vi "S8300E_RTC_PC_Compare.vi"() -> ()   [LabVIEW 2011]
uses:
  Instance          11 29Saved   Mojo_RTC_SFCS_Compare .vi
  Instance           1 29Saved   Mojo_RTC_SFCS_Compare .vi
  Instance           4 29Saved   Mojo_RTC_SFCS_Compare .vi
  Instance           2 29Saved   Mojo_RTC_SFCS_Compare .vi
panel:
  out "log":string
  out "Temp Log":string
  out "PC_Date_Time":string="15:37"
  out "Tolerance sec":string
  out "UUT sec":i32
  out "UUT min":i32
  out "UUT hour":i32
  out "UUT Day":i32
  out "UUT  Month":i32
  out "UUT Year":i32
  out "UUT-DateTime":string
  out "VISA resource name out":refnum<visa-resource-name>
  out "Start Time":u32
  out "Tolerance_sec_gap":dbl
  out "TimeGap(sec)":dbl format="%#_8f"
  out "sec":i32
  out "minute":i32
  out "hour":i32
  out "day":i32
  out "month":i32
  out "year":i32
  out "PC_Time":string
  out "PC_DATE_STRING":string
  out "STAGE":string
  out "SFCS_IP":string
  # "Error Code:RTC\nError Code:UART"
  # "PC時間與S8300E 時間比較\nPC Time compare to S8300E RTC Time"
  # "2015-6-12"
  # "COM9, Baud 115200"
  # "PC Time:"
  # "UUT-Date-Time:"
  # "Formula :TimeGap=SFCS Time-UUT Time"
  # "<"
  # "Pass Criteria"
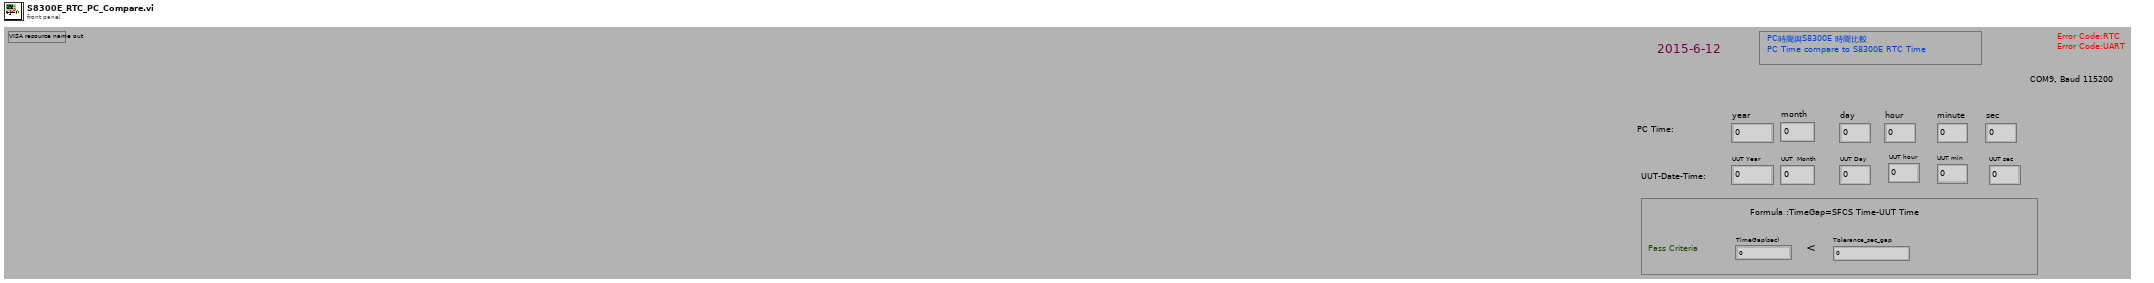
[diagram p1: front panel]
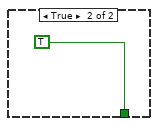
[diagram p5: hidden frame]
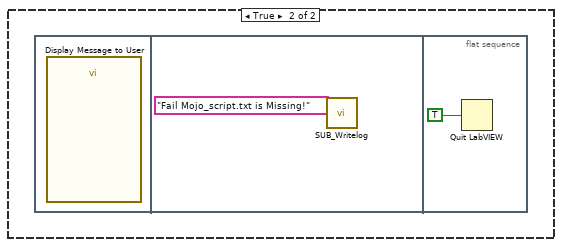
[diagram p7: hidden frame]
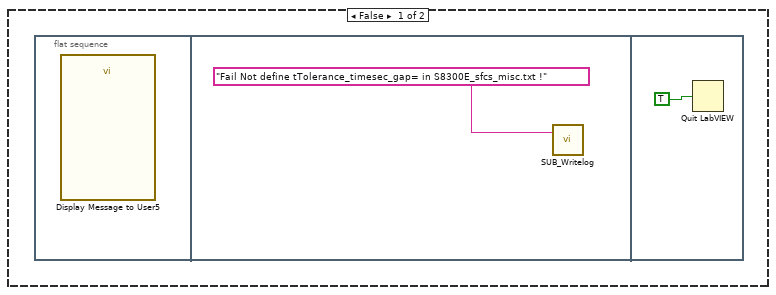
[diagram p8: hidden frame]
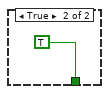
[diagram p11: hidden frame]
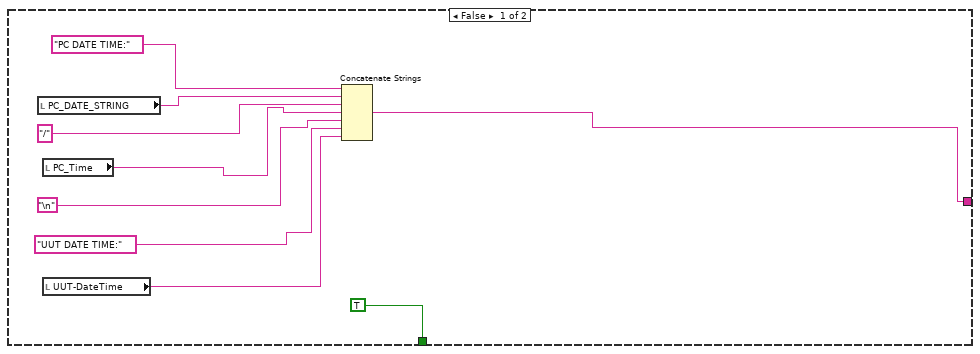
[diagram p12: hidden frame]
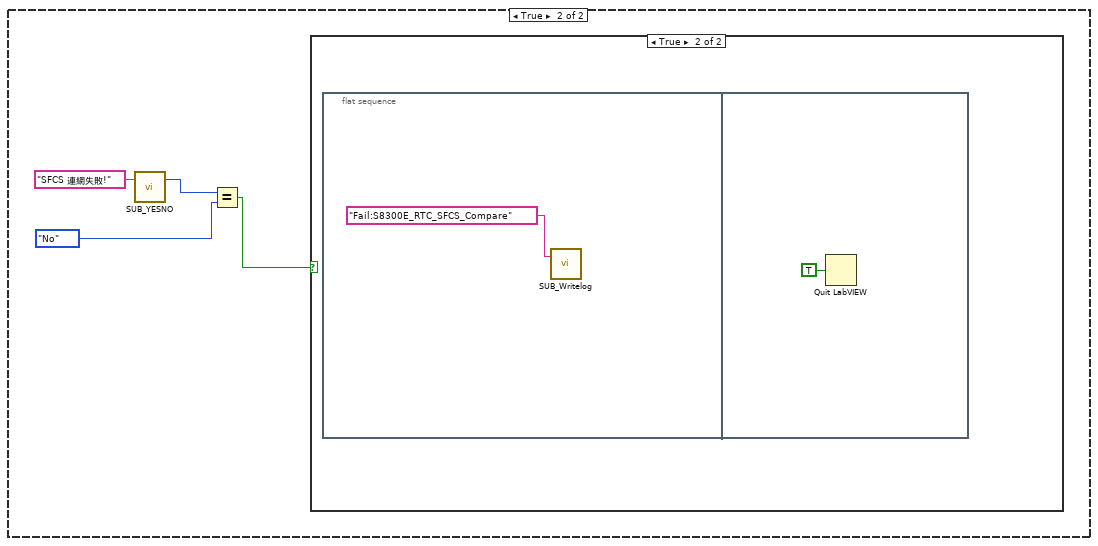
[diagram p14: hidden frame]
diagram:
  n1 = flat-sequence {
    tunnel: [w34] -> w2
    tunnel: w2 -> [w57]
    tunnel: [w57] -> w1
    tunnel: w1 -> [w65]
    frame #0 {
      n2 = Tick Count (ms)() -> (millisecond timer value=→"Start Time":u32)
    }
    frame #1 {
      n3 = call "SUB_COM1_CLOSE.vi"("VISA resource name"=refnum<visa-resource-name> "COM9") -> ()  [unwired: 3 in]
    }
    frame #2 {
      n4 = case shown="True" TRUE {
        frame False {
        }
        frame True {
          n5 = call "SUB_COM9_INIT.vi"("baud rate"=u32 115200) -> ("VISA resource name out"=w9:refnum<visa-resource-name>)  [unwired: 1 in, 1 out]
          "VISA resource name out" <- w9
          n6 = call "SUB_COM1Wrt.vi"("VISA resource name"=w9, "write buffer"="\r") -> ("duplicate VISA resource name"=w6:refnum<visa-resource-name>)  [unwired: 1 in, 1 out]
          n7 = call "SUB_ContinueCom1Read.vi"("Numeric"=1200, "duplicate VISA resource name 2"=w6) -> ()  [unwired: 1 in, 3 out]
        }
      }
    }
    frame #3 {
      n8 = case shown="True" TRUE {
        frame False {
        }
        frame True {
          n9 = while {
            stop <- w19 stop-if-true
            n10 = local read "VISA resource name out"() -> (w18:refnum<visa-resource-name>)
            n11 = Tick Count (ms)() -> (millisecond timer value=w13:u32)
            n12 = call "SUB_COM1Wrt.vi"("VISA resource name"=w18, "write buffer"="\r") -> ("duplicate VISA resource name"=w14:refnum<visa-resource-name>)  [unwired: 1 in, 1 out]
            n13 = call "SUB_READ_COM1_FindString_timeout.vi"("Find this String"="S8300E", "Timeout Seccond"=2.0, "Begin time"=w13, "duplicate VISA resource name 2"=w14) -> ("Output String"=w16:string, "Found String"=w15:bool)  [unwired: 1 in, 1 out]
            n14 = case shown="False" w15 {
              tunnel: w16 -> [w25 _]
              tunnel: [w21 TRUE] -> w19
              frame False {
                n15 = call "SUB_YESNO.vi"("Debug View"=w25, "Status"="UART無正確反應!需有S8300E字串") -> ("yes/no"=w24:enum32{"No Selection", "Yes", "No", "None"})  [unwired: 1 in]
                n16 = Equal?(x=w24, y=enum32{"No Selection", "Yes", "No", "None"}."No") -> (x = y?=w22:bool)
                n17 = case shown="True" w22 {
                  tunnel: [_ w27] -> w21
                  frame False {
                  }
                  frame True {
                    n18 = flat-sequence {
                      tunnel: [w31] -> w27
                      frame #0 {
                        n19 = call "SUB_Writelog.vi"("Pass/Fail"="Fail:S8300E_RTC_SFCS_Compare") -> ()  [unwired: 2 in]
                      }
                      frame #1 {
                        n20 = call "SUB_SFCS_SendResult.vi"("ErrorCode"="UART", "PASS_Fail (1/0)"=i8 0) -> ()  [unwired: 1 out]
                      }
                      frame #2 {
                        w31 = TRUE ("quit? (T)")
                        n21 = Quit LabVIEW(quit? (T)=w31) -> ()
                      }
                    }
                  }
                }
              }
              frame True {
              }
            }
          }
        }
      }
    }
    frame #4 {
      n22 = call "SUB_Read_specifFile.vi"("name or relative path"="S8300E_sfcs_misc.txt" ("Script FileName")) -> ("error out"=w37:errorcluster, "text"=w34:string)  [unwired: 1 in]
      n23 = Unbundle By Name(w37) -> ("code"=w36:i32)
      n24 = Not Equal To 0?(x=w36) -> (x != 0?=w35:bool)
      n25 = case shown="False" w35 {
        tunnel: w34 -> [w38 _]
        frame False {
          n26 = flat-sequence {
            tunnel: w38 -> [w44]
            frame #0 {
              n27 = To Upper Case(1:"SFCS_IP=" ("string")) -> (0:w48:string)
              n28 = To Upper Case(1:w44) -> (0:w49:string)
              n29 = call <vilib>:"Trim Whitespace.vi"("string"=w48) -> ("trimmed string"=w46:string)  [unwired: 1 in]
              n30 = call <vilib>:"Trim Whitespace.vi"("string"=w49) -> ("trimmed string"=w45:string)  [unwired: 1 in]
              n31 = Match Pattern(string=w45, regular expression=w46) -> (after substring=w43:string)  [unwired: 1 in, 3 out]
              n32 = Match Pattern(string=w43, regular expression=";") -> (before substring=w41:string)  [unwired: 1 in, 3 out]
              "SFCS_IP" <- w41
              n33 = Equal?(x=w41, y="") -> (x = y?=w39:bool)
              n34 = case shown="True" w39 {
                frame False {
                }
                frame True {
                  n35 = flat-sequence {
                    frame #0 {
                      n36 = call "Display Message to User2"() -> ()  [unwired: 10 in, 2 out]
                    }
                    frame #1 {
                      n37 = call "SUB_Writelog.vi"("Pass/Fail"="Fail Not Found SFCS_IP=\"xx.xx.xx.xx\" in S8300E_sfcs_misc.txt !") -> ()  [unwired: 2 in]
                    }
                    frame #2 {
                      n38 = Quit LabVIEW(quit? (T)=TRUE) -> ()
                    }
                  }
                }
              }
            }
          }
        }
        frame True {
          n39 = flat-sequence {
            frame #0 {
              n40 = call "Display Message to User"() -> ()  [unwired: 10 in, 2 out]
            }
            frame #1 {
              n41 = call "SUB_Writelog.vi"("Pass/Fail"="Fail Mojo_script.txt is Missing!") -> ()  [unwired: 2 in]
            }
            frame #2 {
              n42 = Quit LabVIEW(quit? (T)=TRUE) -> ()
            }
          }
        }
      }
    }
    frame #5 {
      n43 = call "SUB_FindSpecificString.vi"("Find this String"="Tolerance_timesec_gap=", "String data"=w57) -> ("before \"; \" string"=w54:string, "Found"=w55:bool)  [unwired: 2 in]
      n44 = case shown="True" w55 {
        tunnel: w54 -> [_ w61]
        frame False {
          n45 = flat-sequence {
            frame #0 {
              n46 = call "Display Message to User5"() -> ()  [unwired: 10 in, 2 out]
            }
            frame #1 {
              n47 = call "SUB_Writelog.vi"("Pass/Fail"="Fail Not define tTolerance_timesec_gap= in S8300E_sfcs_misc.txt !") -> ()  [unwired: 2 in]
            }
            frame #2 {
              n48 = Quit LabVIEW(quit? (T)=TRUE) -> ()
            }
          }
        }
        frame True {
          n49 = Fract/Exp String To Number(string=w61) -> (number=→"Tolerance_sec_gap":dbl)  [unwired: 3 in, 1 out]
          "Tolerance sec" <- w61
        }
      }
    }
    frame #6 {
      n50 = To Upper Case(1:"SFCS_STAGE=" ("string")) -> (0:w71:string)
      n51 = To Upper Case(1:w65) -> (0:w72:string)
      n52 = call <vilib>:"Trim Whitespace.vi"("string"=w71) -> ("trimmed string"=w70:string)  [unwired: 1 in]
      n53 = call <vilib>:"Trim Whitespace.vi"("string"=w72) -> ("trimmed string"=w69:string)  [unwired: 1 in]
      n54 = Match Pattern(string=w69, regular expression=w70) -> (after substring=w68:string)  [unwired: 1 in, 3 out]
      n55 = Match Pattern(string=w68, regular expression=";") -> (before substring=w64:string)  [unwired: 1 in, 3 out]
      "STAGE" <- w64
      n56 = Not Equal?(x=w64, y="") -> (x != y?=w62:bool)
      n57 = case shown="False" w62 {
        frame False {
          n58 = flat-sequence {
            frame #0 {
              n59 = call "Display Message to User4"() -> ()  [unwired: 10 in, 2 out]
            }
            frame #1 {
              n60 = call "SUB_Writelog.vi"("Pass/Fail"="Fail :Stage  not define in script file!") -> ()  [unwired: 2 in]
            }
            frame #2 {
              n61 = Quit LabVIEW(quit? (T)=TRUE) -> ()
            }
          }
        }
        frame True {
        }
      }
    }
    frame #7 {
      n62 = while {
        stop <- w80 stop-if-true
        n63 = Concatenate Strings("./rtc.sh -r" ("string"), "\r") -> (w86:string)
        n64 = Tick Count (ms)() -> (millisecond timer value=w76:u32)
        n65 = local read "VISA resource name out"() -> (w84:refnum<visa-resource-name>)
        n66 = call "SUB_COM1Wrt.vi"("VISA resource name"=w84, "write buffer"=w86) -> ("duplicate VISA resource name"=w77:refnum<visa-resource-name>)  [unwired: 1 in, 1 out]
        n67 = call "SUB_READ_COM1_FindString_timeout.vi"("Find this String"="PASSED=", "Timeout Seccond"=3.0, "Begin time"=w76, "duplicate VISA resource name 2"=w77) -> ("Output String"=w79:string)  [unwired: 1 in, 2 out]
        n68 = call "SUB_FindSpecificString.vi"("Find this String"="PASSED=", "String data"=w79) -> ("before \"; \" string"=→"UUT-DateTime":string, "Found"=w81:bool)  [unwired: 2 in]
        n69 = case shown="False" w81 {
          tunnel: w79 -> [w91 _]
          tunnel: [_ TRUE] -> w80
          frame False {
            n70 = call "SUB_YESNO.vi"("Debug View"=w91, "Status"="無法取得UUT RTC Time") -> ("yes/no"=w90:enum32{"No Selection", "Yes", "No", "None"})  [unwired: 1 in]
            n71 = Equal?(x=w90, y=enum32{"No Selection", "Yes", "No", "None"}."No") -> (x = y?=w88:bool)
            n72 = case shown="True" w88 {
              frame False {
              }
              frame True {
                n73 = flat-sequence {
                  frame #0 {
                    n74 = call "SUB_Writelog.vi"("Pass/Fail"="Fail:S8300E_RTC_SFCS_Compare") -> ()  [unwired: 2 in]
                  }
                  frame #1 {
                    n75 = call "SUB_SFCS_SendResult.vi"("ErrorCode"="RTC", "PASS_Fail (1/0)"=i8 0) -> ()  [unwired: 1 out]
                  }
                  frame #2 {
                    n76 = Quit LabVIEW(quit? (T)=TRUE) -> ()
                  }
                }
              }
            }
          }
          frame True {
          }
        }
      }
    }
    frame #8 {
      n77 = local read "UUT-DateTime"() -> (w104:string)
      n78 = call "SUB_UUT_DatTime_Display.vi"("UUT_DateTime_input"=w104) -> ("UUT sec"=→"UUT sec":i32, "UUT min"=→"UUT min":i32, "UUT hour"=→"UUT hour":i32, "UUT Day"=→"UUT Day":i32, "UUT  Month"=→"UUT  Month":i32, "UUT Year"=→"UUT Year":i32)
    }
    frame #9 {
      n79 = while {
        shift-right: [w109] -> w105
        shift-left: "" -> [w107]
        stop <- w111 stop-if-true
        n80 = call "SUB_GETDateTime_String.vi"() -> ("date/time string"=w110:string)  [unwired: 3 in]
        "PC_Date_Time" <- w110
        n81 = To Upper Case(1:"FAIL" ("string")) -> (0:w118:string)
        n82 = To Upper Case(1:"NG" ("string")) -> (0:w126:string)
        n83 = To Upper Case(1:w110) -> (0:w127:string)
        n84 = call <vilib>:"Trim Whitespace.vi"("string"=w118) -> ("trimmed string"=w115:string)  [unwired: 1 in]
        n85 = call <vilib>:"Trim Whitespace.vi"("string"=w126) -> ("trimmed string"=w123:string)  [unwired: 1 in]
        n86 = call <vilib>:"Trim Whitespace.vi"("string"=w127) -> ("trimmed string"=w119:string)  [unwired: 1 in]
        n87 = Match Pattern(string=w110, regular expression=" ") -> (before substring=w121:string, after substring=w120:string)  [unwired: 1 in, 2 out]
        n88 = Match Pattern(string=w119, regular expression=w123) -> (match substring=w124:string)  [unwired: 1 in, 3 out]
        n89 = Match Pattern(string=w119, regular expression=w115) -> (match substring=w116:string)  [unwired: 1 in, 3 out]
        n90 = Equal?(x=w116, y=w115) -> (x = y?=w113:bool)
        n91 = Equal?(x=w124, y=w123) -> (x = y?=w114:bool)
        n92 = Or(x=w114, y=w113) -> (x .or. y?=w112:bool)
        n93 = case shown="False" w112 {
          tunnel: w121 -> [w141 _]
          tunnel: w120 -> [w140 _]
          tunnel: [w135 _] -> w111
          tunnel: [w128 _] -> w108
          frame False {
            n94 = flat-sequence {
              tunnel: w141 -> [w144]
              tunnel: w140 -> [w142]
              tunnel: [w148] -> w133
              tunnel: [w147] -> w131
              tunnel: [w146] -> w129
              tunnel: [w166] -> w139
              tunnel: [w165] -> w138
              tunnel: [w164] -> w137
              tunnel: [w163] -> w134
              tunnel: w133 -> [w163]
              tunnel: [w162] -> w132
              tunnel: w131 -> [w162]
              tunnel: [w161] -> w130
              tunnel: w129 -> [w161]
              tunnel: w139 -> [w181]
              tunnel: w138 -> [w180]
              tunnel: w137 -> [w179]
              tunnel: [w186] -> w136
              tunnel: w134 -> [w184]
              tunnel: w132 -> [w183]
              tunnel: w130 -> [w182]
              tunnel: w136 -> [w191]
              tunnel: [w188] -> w135
              tunnel: [w187] -> w128
              frame #0 {
                n95 = call <vilib>:"Trim Whitespace.vi"("string"=w144) -> ("trimmed string"=→"PC_DATE_STRING":string)  [unwired: 1 in]
                n96 = call <vilib>:"Trim Whitespace.vi"("string"=w142) -> ("trimmed string"=→"PC_Time":string)  [unwired: 1 in]
              }
              frame #1 {
                w155 = "/" ("regular expression")
                n97 = local read "PC_DATE_STRING"() -> (w160:string)
                n98 = Match Pattern(string=w160, regular expression=w155) -> (before substring=w159:string, after substring=w156:string)  [unwired: 1 in, 2 out]
                n99 = Match Pattern(string=w156, regular expression=w155) -> (before substring=w152:string, after substring=w150:string)  [unwired: 1 in, 2 out]
                n100 = call <vilib>:"Trim Whitespace.vi"("string"=w159) -> ("trimmed string"=w158:string)  [unwired: 1 in]
                n101 = To Upper Case(1:w158) -> (0:w157:string)
                n102 = call <vilib>:"Trim Whitespace.vi"("string"=w150) -> ("trimmed string"=w151:string)  [unwired: 1 in]
                n103 = call <vilib>:"Trim Whitespace.vi"("string"=w152) -> ("trimmed string"=w154:string)  [unwired: 1 in]
                n104 = To Upper Case(1:w151) -> (0:w149:string)
                n105 = To Upper Case(1:w154) -> (0:w153:string)
                n106 = Decimal String To Number(string=w157) -> (number=w148:i32)  [unwired: 2 in, 1 out]
                "year" <- w148
                n107 = Decimal String To Number(string=w149) -> (number=w146:i32)  [unwired: 2 in, 1 out]
                "day" <- w146
                n108 = Decimal String To Number(string=w153) -> (number=w147:i32)  [unwired: 2 in, 1 out]
                "month" <- w147
              }
              frame #2 {
                w174 = ":" ("regular expression")
                n109 = local read "PC_Time"() -> (w167:string)
                n110 = Match Pattern(string=w167, regular expression=w174) -> (before substring=w178:string, after substring=w175:string)  [unwired: 1 in, 2 out]
                n111 = Match Pattern(string=w175, regular expression=w174) -> (before substring=w171:string, after substring=w169:string)  [unwired: 1 in, 2 out]
                n112 = call <vilib>:"Trim Whitespace.vi"("string"=w178) -> ("trimmed string"=w177:string)  [unwired: 1 in]
                n113 = To Upper Case(1:w177) -> (0:w176:string)
                n114 = call <vilib>:"Trim Whitespace.vi"("string"=w169) -> ("trimmed string"=w170:string)  [unwired: 1 in]
                n115 = call <vilib>:"Trim Whitespace.vi"("string"=w171) -> ("trimmed string"=w173:string)  [unwired: 1 in]
                n116 = To Upper Case(1:w170) -> (0:w168:string)
                n117 = To Upper Case(1:w173) -> (0:w172:string)
                n118 = Decimal String To Number(string=w176) -> (number=w164:i32)  [unwired: 2 in, 1 out]
                "hour" <- w164
                n119 = Decimal String To Number(string=w168) -> (number=w166:i32)  [unwired: 2 in, 1 out]
                "sec" <- w166
                n120 = Decimal String To Number(string=w172) -> (number=w165:i32)  [unwired: 2 in, 1 out]
                "minute" <- w165
              }
              frame #3 {
                n121 = local read "UUT-DateTime"() -> (w185:string)
                n122 = call "SUB_TimeGAP_SFCS_RTC.vi"("SFCS year"=w184, "UUT_DateTime_input"=w185, "SFCS month"=w183, "SFCS day"=w182, "SFCS hour"=w179, "SFCS minute"=w180, "SFCS second"=w181) -> ("TimeGap(sec)"=w186:dbl)
                "TimeGap(sec)" <- w186
              }
              frame #4 {
                n123 = local read "Tolerance_sec_gap"() -> (w190:dbl)
                n124 = Greater?(x=w191, y=w190) -> (0:w189:bool)
                n125 = case shown="True" w189 {
                  tunnel: [TRUE _] -> w188
                  tunnel: [w192 w201] -> w187
                  frame False {
                    n126 = local read "PC_DATE_STRING"() -> (w198:string)
                    n127 = local read "PC_Time"() -> (w196:string)
                    n128 = local read "UUT-DateTime"() -> (w193:string)
                    n129 = Concatenate Strings("PC DATE TIME:" ("string"), w198, "/" ("string"), w196, "\n", "UUT DATE TIME:" ("string"), w193) -> (w192:string)
                  }
                  frame True {
                    n130 = local read "TimeGap(sec)"() -> (w213:dbl)
                    n131 = local read "Tolerance sec"() -> (w208:string)
                    n132 = Number To Fractional String(number=w213) -> (F-format string=w211:string)  [unwired: 3 in]
                    n133 = Concatenate Strings("Failed:TimeGap 需小於Tolerance Gap", "\n") -> (w204:string)
                    n134 = Concatenate Strings("目前TimeGap=" ("string"), w211, "\n", "目前ToleranceGap=" ("string"), w208) -> (w203:string)
                    n135 = call "SUB_YESNO.vi"("Debug View"=w203, "Status"=w204) -> ("yes/no"=w207:enum32{"No Selection", "Yes", "No", "None"})  [unwired: 1 in]
                    n136 = Concatenate Strings(w204, w203) -> (w202:string)
                    n137 = Equal?(x=w207, y=enum32{"No Selection", "Yes", "No", "None"}."No") -> (x = y?=w205:bool)
                    n138 = case shown="True" w205 {
                      tunnel: [w216 w217] -> w201
                      tunnel: w202 -> [w216 w217]
                      frame False {
                      }
                      frame True {
                        n139 = flat-sequence {
                          frame #0 {
                            n140 = local read "Temp Log"() -> (w218:string)
                            n141 = Concatenate Strings("Fail:S8300E_RTC_SFCS_Compare" ("Pass/Fail"), "\n", w218) -> (w221:string)
                            n142 = call "SUB_Writelog.vi"("Pass/Fail"=w221) -> ()  [unwired: 2 in]
                          }
                          frame #1 {
                            n143 = call "SUB_SFCS_SendResult.vi"("ErrorCode"="RTC", "PASS_Fail (1/0)"=i8 0) -> ()  [unwired: 1 out]
                          }
                          frame #2 {
                            n144 = Quit LabVIEW(quit? (T)=TRUE) -> ()
                          }
                        }
                      }
                    }
                  }
                }
              }
            }
          }
          frame True {
            n145 = call "SUB_YESNO.vi"("Status"="SFCS 連網失敗!") -> ("yes/no"=w227:enum32{"No Selection", "Yes", "No", "None"})  [unwired: 2 in]
            n146 = Equal?(x=w227, y=enum32{"No Selection", "Yes", "No", "None"}."No") -> (x = y?=w225:bool)
            n147 = case shown="True" w225 {
              frame False {
              }
              frame True {
                n148 = flat-sequence {
                  frame #0 {
                    n149 = call "SUB_Writelog.vi"("Pass/Fail"="Fail:S8300E_RTC_SFCS_Compare") -> ()  [unwired: 2 in]
                  }
                  frame #1 {
                    n150 = Quit LabVIEW(quit? (T)=TRUE) -> ()
                  }
                }
              }
            }
          }
        }
        n151 = Concatenate Strings(w107, w108) -> (w109:string)
        "Temp Log" <- w109
      }
      "log" <- w105
    }
    frame #10 {
      n152 = call "SUB_COM1_CLOSE.vi"("VISA resource name"=refnum<visa-resource-name> "COM9") -> ()  [unwired: 3 in]
    }
    frame #11 {
      w237 = "***Not Good ***" ("replace string (\"\")")
      w233 = "\r"
      n153 = local read "PC_Date_Time"() -> (w241:string)
      n154 = local read "TimeGap(sec)"() -> (w244:dbl)
      n155 = local read "log"() -> (w232:string)
      n156 = local read "UUT-DateTime"() -> (w246:string)
      n157 = Tick Count (ms)() -> (millisecond timer value=w250:u32)
      n158 = local read "Start Time"() -> (w249:u32)
      n159 = call "SUB_CAL_TESTTIME.vi"("Test Item name"="S8300E_RTC_SFCS_Compare", "Stop tick time"=w250, "Start tick time"=w249) -> ("Test Time output"=w242:string)  [unwired: 2 in]
      n160 = Number To Fractional String(number=w244) -> (F-format string=w243:string)  [unwired: 3 in]
      n161 = Concatenate Strings("Pass :S8300E_RTC_SFCS_Compare" ("Pass/Fail"), w233, w232, w233, "Message From Local PC Time:", w241, w233, "Message From UUT:", w246, w233, "TimeGap=", w243, w233, w242) -> (w235:string)
      n162 = call "SUB_SEARCH_REPLACE_STR.vi"("replace string (\"\")"=w237, "search string"="FAILED", "input string"=w235) -> ("result string"=w239:string)  [unwired: 2 in]
      n163 = call "SUB_SEARCH_REPLACE_STR.vi"("replace string (\"\")"=w237, "search string"="FAIL", "input string"=w239) -> ("result string"=w236:string)  [unwired: 2 in]
      n164 = call "SUB_Writelog.vi"("Pass/Fail"=w236) -> ()  [unwired: 2 in]
    }
    frame #12 {
      n165 = Request Deallocation(TRUE ("flag")) -> ()
    }
    frame #13 {
      n166 = Quit LabVIEW(quit? (T)=TRUE) -> ()
    }
  }
